vi "Строку в коор. выстрела лазера (SubVI).vi"(12 "Строка числовых параметров мишеней":string) -> (22 "Положение XY лазера":cluster{i32, i32}, 25 "Положение информации о выстреле":cluster{i32, i32})   [LabVIEW 2013]
doc: "преобразование строки чисел параметров мишени в координаты позиции лазера и информации о выстреле"
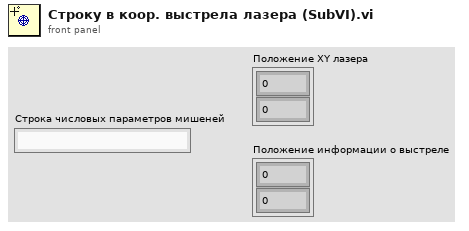
[diagram p1: front panel]
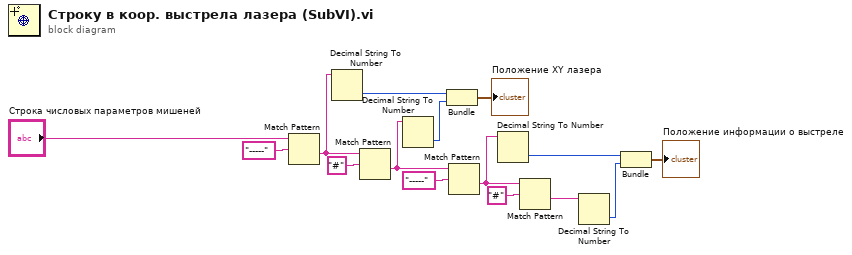
[diagram p0: block diagram]
diagram:
  n1 = Match Pattern(string="Строка числовых параметров мишеней", regular expression="-----") -> (after substring=w4:string)  [unwired: 1 in, 3 out]
  n2 = Decimal String To Number(string=w4) -> (number=w13:i32)  [unwired: 2 in, 1 out]
  n3 = Match Pattern(string=w4, regular expression="#") -> (after substring=w9:string)  [unwired: 1 in, 3 out]
  n4 = Decimal String To Number(string=w9) -> (number=w12:i32)  [unwired: 2 in, 1 out]
  n5 = Bundle(w13, w12) -> (→"Положение XY лазера":cluster{i32, i32})  [unwired: 1 in]
  n6 = Match Pattern(string=w9, regular expression="-----") -> (after substring=w6:string)  [unwired: 1 in, 3 out]
  n7 = Decimal String To Number(string=w6) -> (number=w15:i32)  [unwired: 2 in, 1 out]
  n8 = Match Pattern(string=w6, regular expression="#") -> (after substring=w5:string)  [unwired: 1 in, 3 out]
  n9 = Decimal String To Number(string=w5) -> (number=w14:i32)  [unwired: 2 in, 1 out]
  n10 = Bundle(w15, w14) -> (→"Положение информации о выстреле":cluster{i32, i32})  [unwired: 1 in]
